vi "WM Significant Wave Height.vi"(1 "Input":dbl[](array[numeric]) format="%.2f") -> (0 "Significant Wave Height":dbl format="%.2f")   [LabVIEW 2012]
uses:
  <vilib>/Analysis/NI_AALBase.lvlib
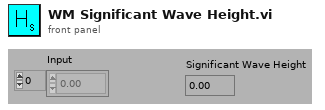
[diagram p1: front panel]
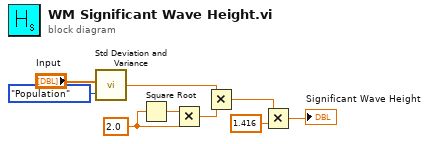
[diagram p0: block diagram]
diagram:
  w8 = 2.0 ("y")
  n1 = call <vilib>:"Std Deviation and Variance.vi"("X"="Input", "Weighting (Sample)"=enum16{"Sample", "Population"}."Population") -> ("standard deviation"=w5:dbl)  [unwired: 2 out]
  n2 = Square Root(x=w8) -> (sqrt(x)=w7:dbl)
  n3 = Multiply(x=w7, y=w8) -> (x*y=w6:dbl)
  n4 = Multiply(x=w5, y=w6) -> (x*y=w4:dbl)
  n5 = Multiply(x=w4, y=1.416) -> (x*y=→"Significant Wave Height":dbl)
